vi "test - Populate Variant with Unsigned Integer.vi"(8 "error in (no error)":errorcluster, 11 "TestCase in":refnum<class "Python Data Tools Tests.lvclass">) -> (0 "error out":errorcluster, 3 "TestCase out":refnum<class "Python Data Tools Tests.lvclass">)   [LabVIEW 2020, in "Python Data Tools Tests.lvclass"]
uses:
  Python Data Tools Tests.lvclass
  Python Data Tools Tests.lvclass/Python Data Tools Tests.ctl
  <vilib>/addons/_JKI Toolkits/VI Tester/TestCase.llb/TestCase.lvclass
  source/jki_python_data_tools.lvlib
  C:/Program Files/National Instruments/LabVIEW 2020/vi.lib/addons/_JKI Toolkits/VI Tester/TestCase.llb/TestCase.lvclass
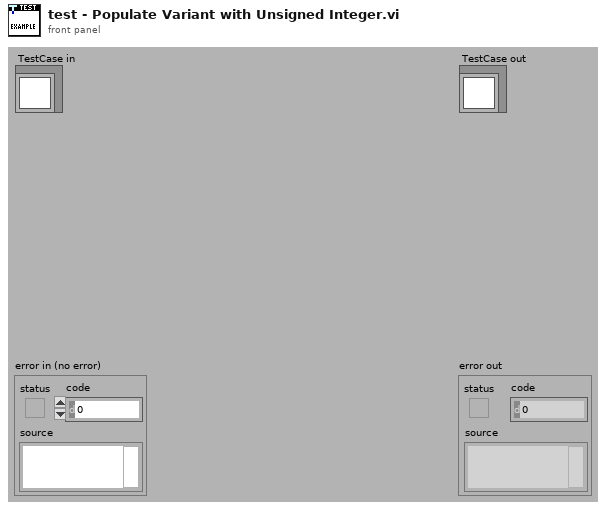
[diagram p1: front panel]
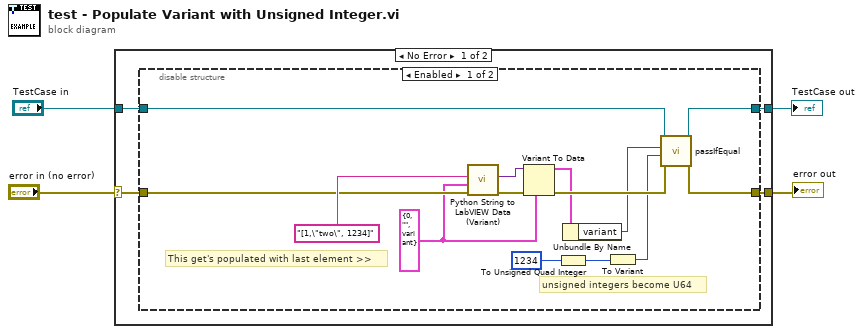
[diagram p0: block diagram]
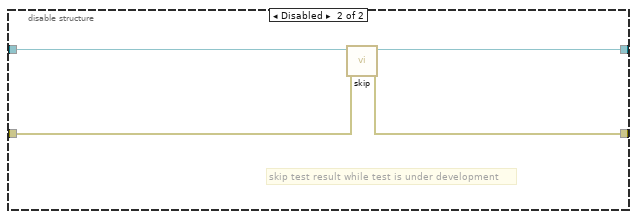
[diagram p2: hidden frame]
diagram:
  n1 = case shown="No Error" "error in (no error)" {
    selector: "error in (no error)" -> [w6 w28]
    tunnel: [w5 w28] -> w3
    tunnel: [w7 w27] -> w1
    tunnel: "TestCase in" -> [w8 w27]
    frame No Error {
      n2 = disable-structure shown="Enabled" {
        disable-tunnel: w8 -> [w22 w26]
        disable-tunnel: [w21 w23] -> w7
        disable-tunnel: w6 -> [w15 w25]
        disable-tunnel: [w20 w24] -> w5
        frame Enabled {
          w14 = cluster{i32, string, "variant":variant} {0, "", "variant"=variant}
          # "unsigned integers become U64"
          # "This get's populated with last element >>"
          n3 = call "Python String to LabVIEW Data (Variant).vi"("error in (no error)"=w15, "type"=w14, "Python String"="[1,\"two\", 1234]") -> ("error out"=w17:errorcluster, "LabVIEW Data"=w18:variant)  [unwired: 7 in]
          n4 = Variant To Data(error in=w17, type=w14, Variant=w18) -> (data=w12:cluster{i32, string, "variant":variant}, error out=w16:errorcluster)
          n5 = To Unsigned Quad Integer(1:1234) -> (0:w9:u64)
          n6 = Unbundle By Name(w12) -> ("variant"=w13:variant)
          n7 = To Variant(anything=w9) -> (Variant=w11:variant)
          n8 = call-dynamic "passIfEqual.vi"("error in (no error)"=w16, "y"=w11, "x"=w13, "TestCase in"=w22) -> ("error out"=w20:errorcluster, "TestCase out"=w21:refnum<class "Python Data Tools Tests.lvclass">)  [unwired: 6 in]
        }
        frame Disabled {
          # "skip test result while test is under development"
          n9 = call <vilib>:"skip.vi"("error in (no error)"=w25, "TestCase in"=w26) -> ("error out"=w24:errorcluster, "TestCase out"=w23:refnum<class "Python Data Tools Tests.lvclass">)  [unwired: 8 in]
        }
      }
    }
    frame Error {
    }
  }
  "error out" <- w3
  "TestCase out" <- w1
